vi "user maped buttons.vi"(3 "previous button state":u32, 4 "gp button info":T2, 5 "map references":T3) -> (0 "current button state":u32, 1 "mapped gp buttons":T1)   [LabVIEW 2012]
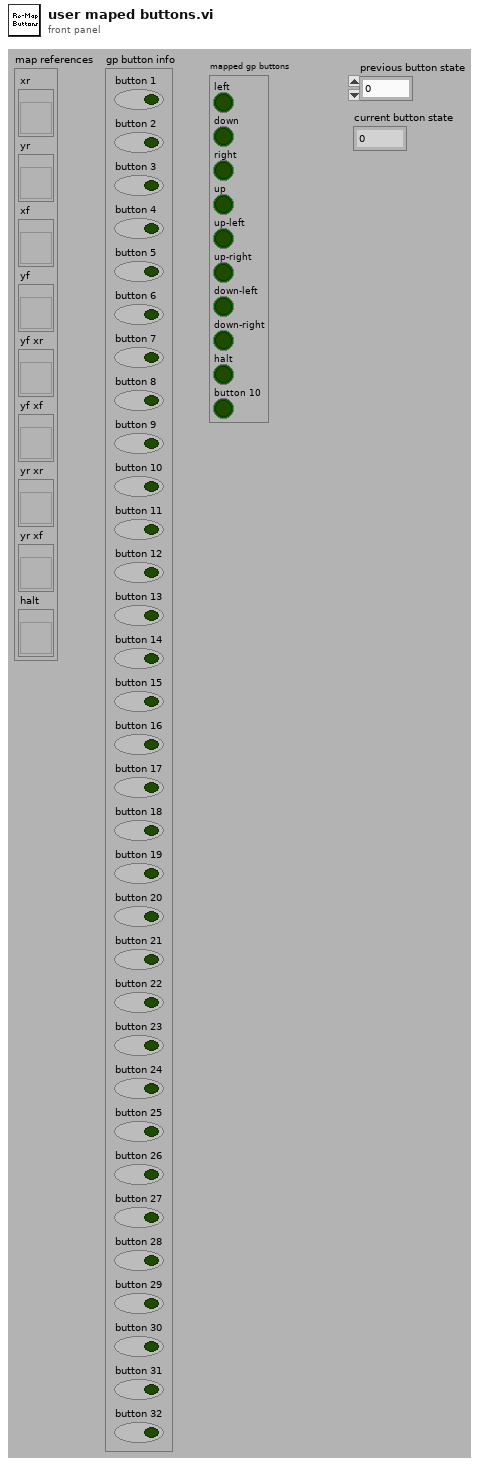
[diagram p1: front panel]
types:
  T1 = cluster{"left":bool, "down":bool, "right":bool, "up":bool, "up-left":bool, "up-right":bool, "down-left":bool, "down-right":bool, "halt":bool, "button 10":bool}
  T2 = cluster{"button 1":bool, "button 2":bool, "button 3":bool, "button 4":bool, "button 5":bool, "button 6":bool, "button 7":bool, "button 8":bool, "button 9":bool, "button 10":bool, "button 11":bool, "button 12":bool, "button 13":bool, "button 14":bool, "button 15":bool, "button 16":bool, "button 17":bool, "button 18":bool, "button 19":bool, "button 20":bool, "button 21":bool, "button 22":bool, "button 23":bool, "button 24":bool, "button 25":bool, "button 26":bool, "button 27":bool, "button 28":bool, "button 29":bool, "button 30":bool, "button 31":bool, "button 32":bool}
  T3 = cluster{"xr":refnum<vi>, "yr":refnum<vi>, "xf":refnum<vi>, "yf":refnum<vi>, "yf xr":refnum<vi>, "yf xf":refnum<vi>, "yr xr":refnum<vi>, "yr xf":refnum<vi>, "halt":refnum<vi>}
  T4 = cluster{"[0]":bool, "[1]":bool, "[2]":bool, "[3]":bool, "[4]":bool, "[5]":bool, "[6]":bool, "[7]":bool, "[8]":bool}
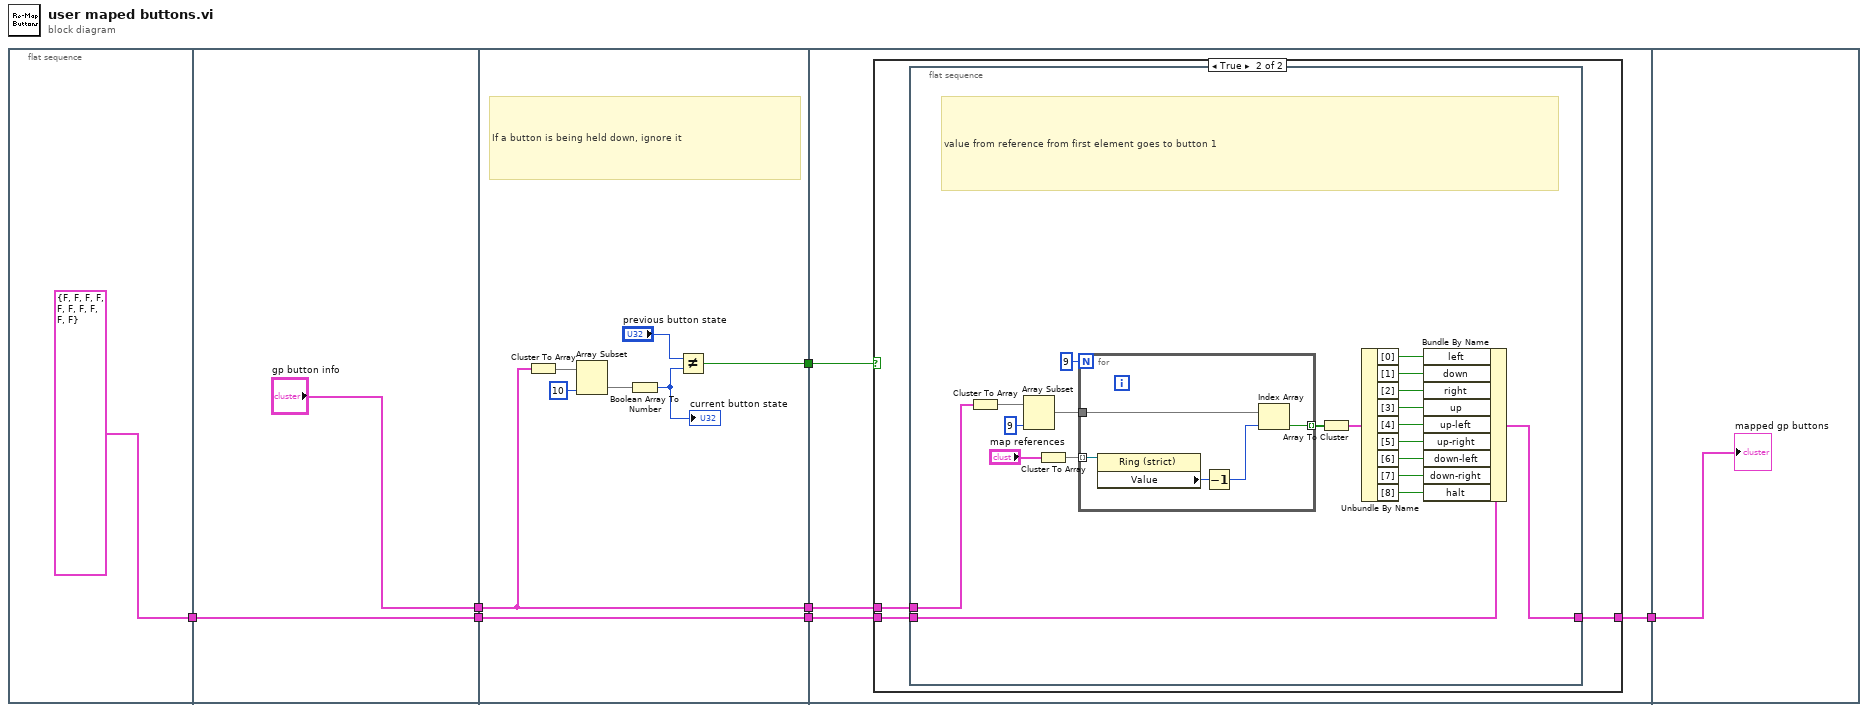
[diagram p0: block diagram]
diagram:
  n1 = flat-sequence {
    tunnel: [T1 {"left"=FALSE, "down"=FALSE, "right"=FALSE, "up"=FALSE, "up-left"=FALSE, "up-right"=FALSE, "down-left"=FALSE, "down-right"=FALSE, "halt"=FALSE, "button 10"=FALSE} ("button info")] -> w4
    tunnel: ["gp button info"] -> w7
    tunnel: w4 -> [w9]
    tunnel: [w9] -> w2
    tunnel: w7 -> [w12]
    tunnel: [w12] -> w6
    tunnel: [w13] -> w5
    tunnel: [w11] -> w3
    tunnel: w2 -> [w11]
    tunnel: w6 -> [w22]
    tunnel: w5 -> [w21]
    tunnel: w3 -> [w20]
    tunnel: [w19] -> w1
    tunnel: w1 -> [w52]
    frame #0 {
    }
    frame #1 {
    }
    frame #2 {
      # "If a button is being held down, ignore it"
      n2 = Cluster To Array(cluster=w12) -> (array=w14:bool[])
      n3 = Array Subset(array=w14, length=10) -> (w16:bool[])  [unwired: 1 in]
      n4 = Boolean Array To Number(Boolean array=w16) -> (number=w17:u32)
      "current button state" <- w17
      n5 = Not Equal?(x="previous button state", y=w17) -> (x != y?=w13:bool)
    }
    frame #3 {
      n6 = case shown="True" w21 {
        tunnel: w22 -> [_ w26]
        tunnel: w20 -> [w23 w25]
        tunnel: [w23 w24] -> w19
        frame False {
        }
        frame True {
          n7 = flat-sequence {
            tunnel: [w45] -> w24
            tunnel: w25 -> [w46]
            tunnel: w26 -> [w36]
            frame #0 {
              # "value from reference from first element goes to button 1"
              n8 = Cluster To Array(cluster=w36) -> (array=w42:bool[])
              n9 = Array Subset(array=w42, length=9) -> (w41:bool[])  [unwired: 1 in]
              n10 = Cluster To Array(cluster="map references") -> (array=w37:refnum<vi>[])
              n11 = for {
                N: 9 -> [_]
                tunnel: w37 -> [w51] mode=indexing
                tunnel: w41 -> [w50]
                tunnel: [w47] -> w40 mode=indexing
                n12 = property on="Property Node" class="Ring (strict)"(reference=w51) -> ("Value"=w49:u16)  [unwired: 1 in, 2 out]
                n13 = Decrement(x=w49) -> (x-1=w48:u16)
                n14 = Index Array(array=w50, index=w48) -> (element=w47:bool)
              }
              n15 = Array To Cluster(array=w40) -> (cluster=w44:T4)
              n16 = Unbundle By Name(w44) -> ("[0]"=w35:bool, "[1]"=w34:bool, "[2]"=w33:bool, "[3]"=w32:bool, "[4]"=w31:bool, "[5]"=w30:bool, "[6]"=w29:bool, "[7]"=w28:bool, "[8]"=w27:bool)
              n17 = Bundle By Name(cluster=w46, "left"=w35, "down"=w34, "right"=w33, "up"=w32, "up-left"=w31, "up-right"=w30, "down-left"=w29, "down-right"=w28, "halt"=w27) -> (w45:T1)
            }
          }
        }
      }
    }
    frame #4 {
      "mapped gp buttons" <- w52
    }
  }
